vi "TSCAN_GetSignalValue_CANFD.vi"(6 "All_ID":i32[](array[numeric]) format="%x", 7 "TLIBCANFD":T1, 8 "错误输入（无错误）":errorcluster, 9 "ALLSignalName":string[][](array[string]), 10 "ALLMessage":string[](array[string]), 11 "路径输入":path) -> (0 "错误输出":errorcluster, 1 "SigValue":dbl[](array[numeric]), 2 "SigName":string[](array[string]), 3 "路径输出":path, 4 "Message Name":string[](array[string]))   [LabVIEW 2014]
panel:
  out "Element index":i32
  out "tsdb_load_can_db":i32
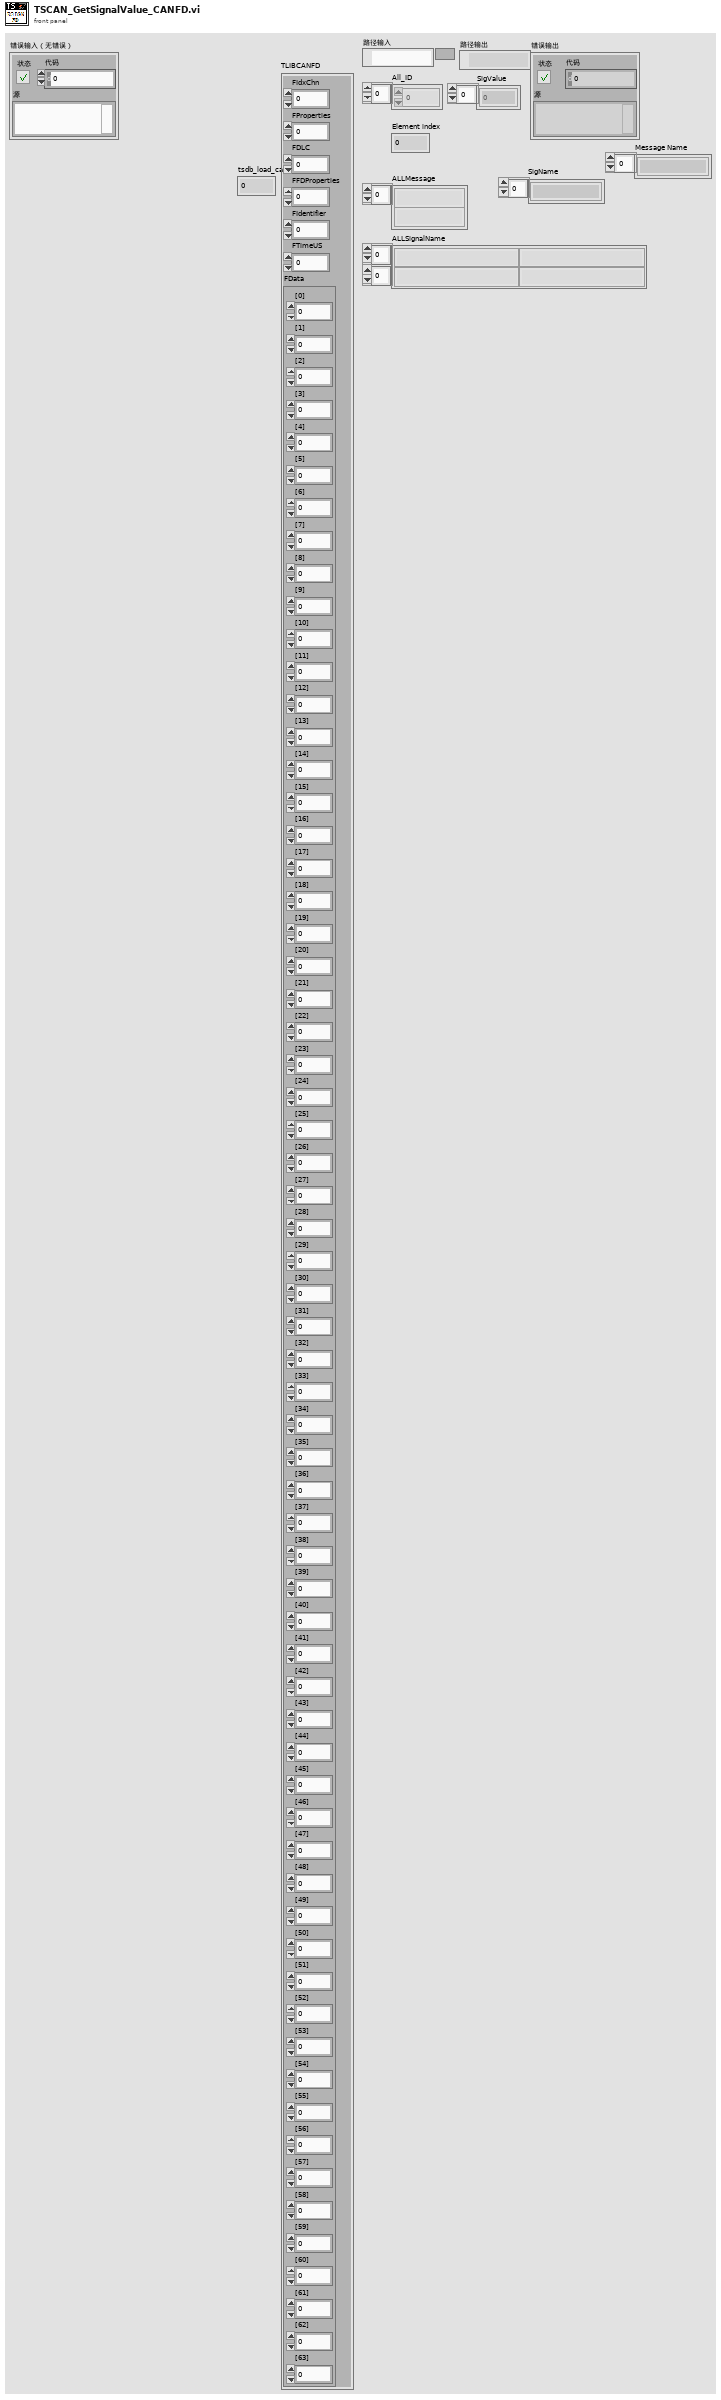
[diagram p1: front panel]
types:
  T1 = cluster{"FIdxChn":u8, "FProperties":u8, "FDLC":u8, "FFDProperties":u8, "FIdentifier":i32, "FTimeUS":u64, "FData":cluster{"[0]":u8, "[1]":u8, "[2]":u8, "[3]":u8, "[4]":u8, "[5]":u8, "[6]":u8, "[7]":u8, "[8]":u8, "[9]":u8, "[10]":u8, "[11]":u8, "[12]":u8, "[13]":u8, "[14]":u8, "[15]":u8, "[16]":u8, "[17]":u8, "[18]":u8, "[19]":u8, "[20]":u8, "[21]":u8, "[22]":u8, "[23]":u8, "[24]":u8, "[25]":u8, "[26]":u8, "[27]":u8, "[28]":u8, "[29]":u8, "[30]":u8, "[31]":u8, "[32]":u8, "[33]":u8, "[34]":u8, "[35]":u8, "[36]":u8, "[37]":u8, "[38]":u8, "[39]":u8, "[40]":u8, "[41]":u8, "[42]":u8, "[43]":u8, "[44]":u8, "[45]":u8, "[46]":u8, "[47]":u8, "[48]":u8, "[49]":u8, "[50]":u8, "[51]":u8, "[52]":u8, "[53]":u8, "[54]":u8, "[55]":u8, "[56]":u8, "[57]":u8, "[58]":u8, "[59]":u8, "[60]":u8, "[61]":u8, "[62]":u8, "[63]":u8}}
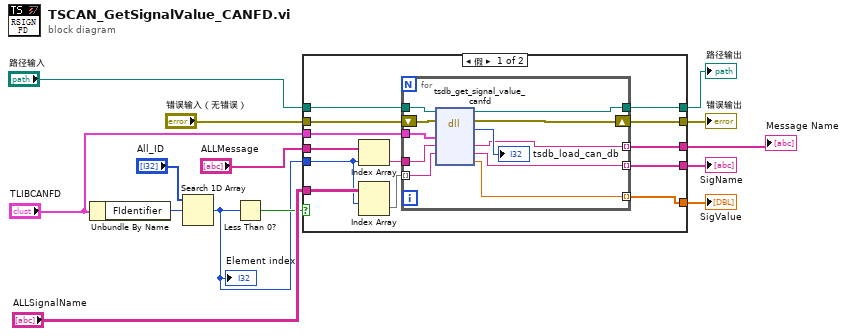
[diagram p0: block diagram]
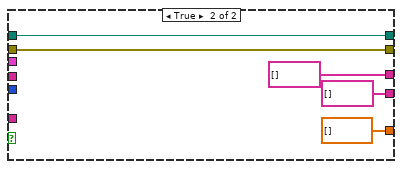
[diagram p2: hidden frame]
diagram:
  n1 = Unbundle By Name("TLIBCANFD") -> ("FIdentifier"=w13:i32)
  n2 = Search 1D Array(1D array="All_ID", element=w13) -> (index of element=w2:i32)  [unwired: 1 in]
  "Element index" <- w2
  n3 = Less Than 0?(x=w2) -> (x < 0?=w3:bool)
  n4 = case shown="假" w3 {
    tunnel: "ALLMessage" -> [w27 _]
    tunnel: "ALLSignalName" -> [w25 _]
    tunnel: w2 -> [w24 _]
    tunnel: [w22 dbl[] []] -> w10
    tunnel: [w21 string[] []] -> w9
    tunnel: "错误输入（无错误）" -> [w20 w41]
    tunnel: [w19 w41] -> w7
    tunnel: "路径输入" -> [w18 w40]
    tunnel: [w17 w40] -> w5
    tunnel: "TLIBCANFD" -> [w16 _]
    tunnel: [w15 string[] []] -> w1
    frame False {
      n5 = Index Array(array=w27, index=w24) -> (element=w26:string)
      n6 = Index Array(array=w25, index (row)=w24) -> (element=w23:string[])  [unwired: 1 in]
      n7 = for {
        tunnel: w16 -> [w38]
        tunnel: w26 -> [w37]
        tunnel: w23 -> [w35] mode=indexing
        tunnel: [w34] -> w22 mode=indexing
        tunnel: [w33] -> w21 mode=indexing
        tunnel: w18 -> [w30]
        tunnel: [w29] -> w17
        shift-right: [w31] -> w19
        shift-left: w20 -> [w32]
        tunnel: [w28] -> w15 mode=indexing
        n8 = dll-call lib="D:/Program Files (x86)/TOSUN/TSMaster/bin/TSMaster.dll" fn="tsdb_get_signal_value_canfd"(path in=w30, error in=w32, "CANObJ"=w38, "Message"=w37, "Signal"=w35) -> (path out=w29:path, error out=w31:errorcluster, "tsdb_get_signal_value_can"=→"tsdb_load_can_db":i32, "Message"=w28:string, "Signal"=w33:string, "SigValue"=w34:dbl)  [unwired: 3 in]
      }
    }
    frame True {
    }
  }
  "SigValue" <- w10
  "SigName" <- w9
  "错误输出" <- w7
  "路径输出" <- w5
  "Message Name" <- w1
